vi "Reserve UART.vi"(7 "UART Pins":T1={"TX GPIO"=-1, "RX GPIO"=-1}, 8 "error in (no error)":errorcluster, 9 "Purpose":string, 10 "UART #":T3=-1, 11 "Session in":refnum<class "Session.lvclass">) -> (0 "error out":errorcluster, 3 "Session out":refnum<class "Session.lvclass">)   [LabVIEW 2024, in "CTI.lvlib" / "Session.lvclass"]
uses:
  Session.lvclass
  UART Number.ctl
  UART Pins.ctl
  GPIO Number.ctl
  Resource/Resource.lvclass/Resource.ctl
  Session.lvclass/Session.ctl
  dcef0d26-6755-4235-b060-6b0e00c3d74f.vi
  dcef0d26-6755-4235-b060-6b0e00c3d74f.vi/685f7f19-b444-4620-8f66-e6e2ddd64bb8.vi
  UART/UART.lvclass
  C:/Users/nkirchne/Documents/~SANDBOX/Electronics Workflow/build/ForPort/CTI/Resource/Resource.lvclass
  Generate Error.vi
  Resource/Resource.lvclass
  CTI.lvlib
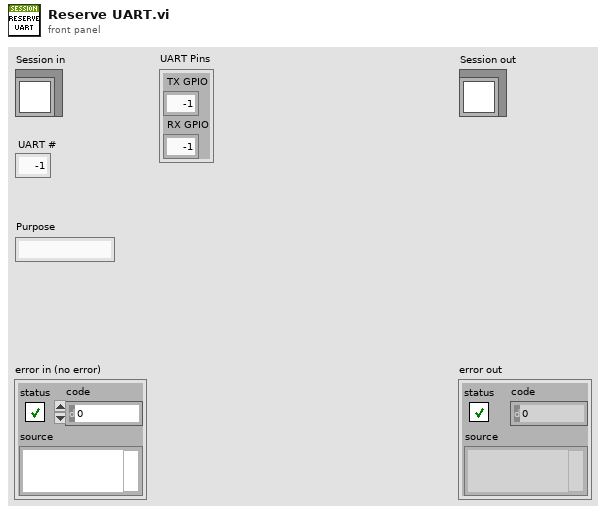
[diagram p1: front panel]
types:
  T1 = typedef "CTI.lvlib/UART Pins.ctl" = cluster{"TX GPIO":T2, "RX GPIO":T2}
  T2 = typedef "CTI.lvlib/GPIO Number.ctl" = i8
  T3 = typedef "CTI.lvlib/UART Number.ctl" = i8
  T4 = typedef "CTI.lvlib/Session.lvclass/Resources.ctl" = cluster{"GPIO":map{T2, refnum<class "GPIO.lvclass">}, "AI":map{T5, refnum<class "AI.lvclass">}, "PWM":map{T2, refnum<class "PWM.lvclass">}, "UART":map{T3, refnum<class "UART.lvclass">}, "I2C":map{T6, refnum<class "I2C.lvclass">}, "SPI":map{T7, refnum<class "SPI.lvclass">}, "SPI CS":map{T2, refnum<class "SPI CS.lvclass">}}
  T5 = typedef "CTI.lvlib/ADC Number.ctl" = i8
  T6 = typedef "CTI.lvlib/I2C Number.ctl" = i8
  T7 = typedef "CTI.lvlib/SPI Number.ctl" = i8
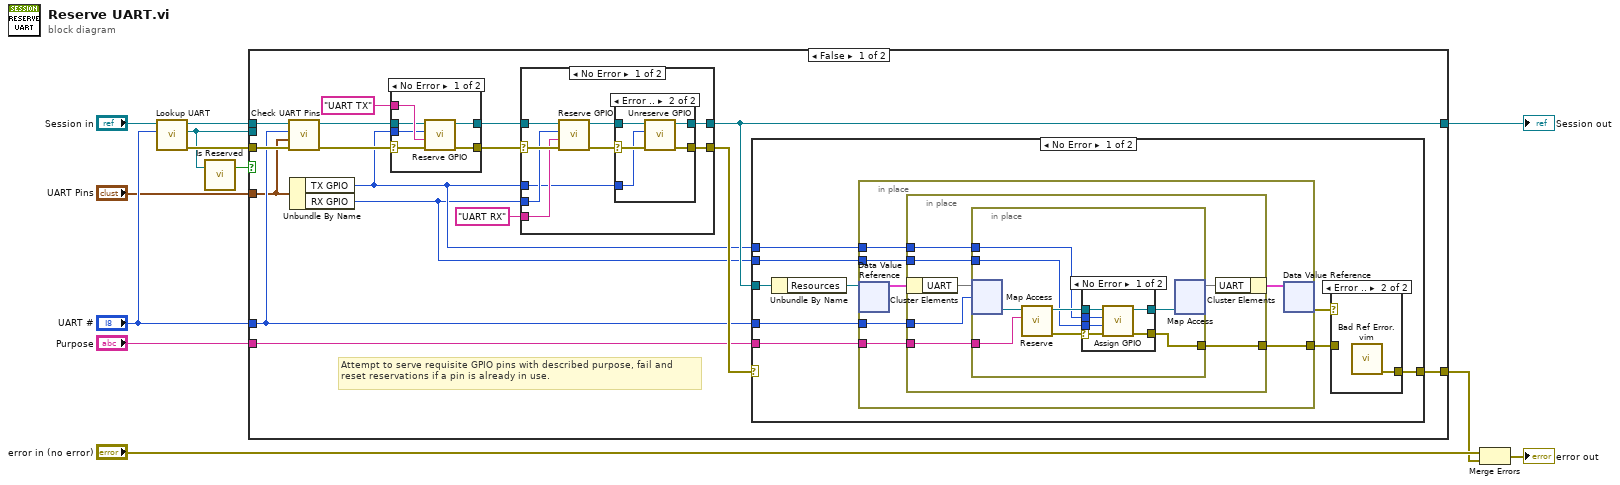
[diagram p0: block diagram]
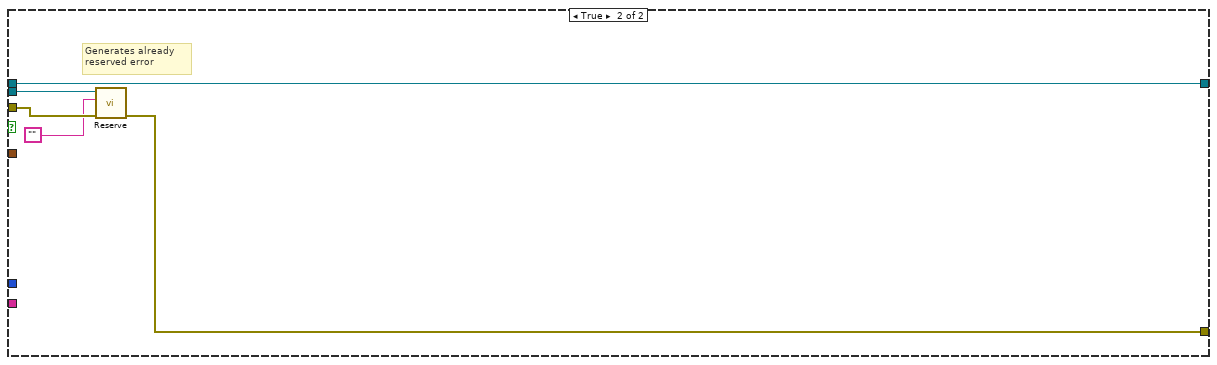
[diagram p8: hidden frame]
diagram:
  n1 = call "Lookup UART.vi"("UART #"="UART #", "Session in"="Session in") -> ("error out"=w12:errorcluster, "UART"=w1:refnum<class "UART.lvclass">, "Session out"=w6:refnum<class "Session.lvclass">)  [unwired: 7 in]
  n2 = call "Is Reserved.vi"("Resource in"=w1) -> ("Reserved"=w2:bool)  [unwired: 6 in]
  n3 = case shown="False" w2 {
    tunnel: w12 -> [w26 w100]
    tunnel: "Purpose" -> [w25 _]
    tunnel: [w24 w98] -> w7
    tunnel: w6 -> [w18 w99]
    tunnel: "UART #" -> [w16 _]
    tunnel: "UART Pins" -> [w15 _]
    tunnel: [w21 w99] -> w3
    tunnel: w1 -> [_ w101]
    frame False {
      # "Attempt to serve requisite GPIO pins with described purpose, fail and reset reservations if a pin is already in use."
      n4 = call "Check UART Pins.vi"("error in (no error)"=w26, "UART Pins"=w15, "UART #"=w16, "Session in"=w18) -> ("error out"=w19:errorcluster, "Session out"=w17:refnum<class "Session.lvclass">)  [unwired: 6 in]
      n5 = Unbundle By Name(w15) -> ("TX GPIO"=w14:T2, "RX GPIO"=w13:T2)
      n6 = case shown="No Error" w19 {
        selector: w19 -> [w30 w36]
        tunnel: [w34 w36] -> w27
        tunnel: "UART TX" ("Purpose") -> [w33 _]
        tunnel: [w32 w35] -> w22
        tunnel: w14 -> [w31 _]
        tunnel: w17 -> [w29 w35]
        frame No Error {
          n7 = call "Reserve GPIO.vi"("error in (no error)"=w30, "Purpose"=w33, "GPIO #"=w31, "Session in"=w29) -> ("error out"=w34:errorcluster, "Session out"=w32:refnum<class "Session.lvclass">)  [unwired: 6 in]
        }
        frame Error {
        }
      }
      n8 = case shown="No Error" w27 {
        selector: w27 -> [w45 w53]
        tunnel: [w38 w53] -> w28
        tunnel: w22 -> [w44 w54]
        tunnel: [w39 w54] -> w21
        tunnel: w13 -> [w43 _]
        tunnel: "UART RX" ("Purpose") -> [w42 _]
        tunnel: w14 -> [w37 _]
        frame No Error {
          n9 = call "Reserve GPIO.vi"("error in (no error)"=w45, "Purpose"=w42, "GPIO #"=w43, "Session in"=w44) -> ("error out"=w41:errorcluster, "Session out"=w40:refnum<class "Session.lvclass">)  [unwired: 6 in]
          n10 = case shown="Error .." w41 {
            selector: w41 -> [w46 w51]
            tunnel: w40 -> [w47 w52]
            tunnel: [w47 w48] -> w39
            tunnel: [w46 w49] -> w38
            tunnel: w37 -> [_ w50]
            frame No Error {
            }
            frame Error {
              n11 = call "Unreserve GPIO.vi"("error in (no error)"=w51, "GPIO #"=w50, "Session in"=w52) -> ("error out"=w49:errorcluster, "Session out"=w48:refnum<class "Session.lvclass">)  [unwired: 7 in]
            }
          }
        }
        frame Error {
        }
      }
      n12 = case shown="No Error" w28 {
        selector: w28 -> [_ w96]
        tunnel: w25 -> [w62 _]
        tunnel: [w59 w96] -> w24
        tunnel: w16 -> [w58 _]
        tunnel: w21 -> [w57 _]
        tunnel: w14 -> [w56 _]
        tunnel: w13 -> [w55 _]
        frame No Error {
          n13 = Unbundle By Name(w57) -> ("Resources"=w63:refnum<data-value>)
          n14 = in-place {
            in-place-border: w58 -> [w70]
            in-place-border: w62 -> [w69]
            in-place-border: [w68] -> w61
            in-place-border: w56 -> [w65]
            in-place-border: w55 -> [w64]
            n15 = in-place-dvr #1(w63) -> (w66:T4)  [unwired: 1 out]
            n16 = in-place {
              in-place-border: w70 -> [w76]
              in-place-border: w69 -> [w75]
              in-place-border: [w74] -> w68
              in-place-border: w65 -> [w72]
              in-place-border: w64 -> [w71]
              n17 = in-place-cluster #2(w66) -> ("UART"=w77:map{T3, refnum<class "UART.lvclass">})
              n18 = in-place {
                in-place-border: w75 -> [w84]
                in-place-border: [w78] -> w74
                in-place-border: w72 -> [w80]
                in-place-border: w71 -> [w79]
                n19 = in-place-map #3(w77, w76) -> (w85:refnum<class "UART.lvclass">)  [unwired: 1 in, 1 out]
                n20 = call "Reserve.vi"("Purpose"=w84, "Resource in"=w85) -> ("error out"=w81:errorcluster, "Resource out"=w83:refnum<class "UART.lvclass">)  [unwired: 8 in]
                n21 = case shown="No Error" w81 {
                  selector: w81 -> [w89 w93]
                  tunnel: w83 -> [w91 w92]
                  tunnel: [w90 w92] -> w82
                  tunnel: w80 -> [w87 _]
                  tunnel: w79 -> [w86 _]
                  tunnel: [w88 w93] -> w78
                  frame No Error {
                    n22 = call "Assign GPIO.vi"("error in (no error)"=w89, "RX"=w86, "TX"=w87, "UART in"=w91) -> ("error out"=w88:errorcluster, "UART out"=w90:refnum<class "UART.lvclass">)  [unwired: 6 in]
                  }
                  frame Error {
                  }
                }
                n23 = in-place-map #3(w82) -> (w73:map{T3, refnum<class "UART.lvclass">})  [unwired: 1 in, 2 out]
              }
              n24 = in-place-cluster #2("UART"=w73) -> (w67:T4)
            }
            n25 = in-place-dvr #1(w67) -> (w60:errorcluster)  [unwired: 1 out]
          }
          n26 = case shown="Error .." w60 {
            tunnel: w61 -> [w94 _]
            tunnel: [w94 w95] -> w59
            frame No Error {
            }
            frame Error {
              n27 = call "Bad Ref Error.vim"() -> ("error out"=w95:errorcluster)  [unwired: 10 in, 1 out]
            }
          }
        }
        frame Error {
          # "Error generated reserving GPIO Pin(s) or looking up I2C #"
        }
      }
    }
    frame True {
      # "Generates already reserved error"
      n28 = call "Reserve.vi"("error in (no error)"=w100, "Purpose"="", "Resource in"=w101) -> ("error out"=w98:errorcluster)  [unwired: 7 in, 1 out]
    }
  }
  "Session out" <- w3
  n29 = Merge Errors("error in (no error)", w7) -> (→"error out":errorcluster)
